vi "GetWindowInfo.vi"(8 "error in (no error)":errorcluster, 11 "Window Title (\"\")":string) -> (0 "error out":errorcluster, 1 "WINDOWINFO":T3 {"dwExStyle" format="%.0x"; "dwStyle" format="%.0x"}, 2 "Active?":bool, 3 "hWnd":T2, 4 "Window data":T1)   [LabVIEW 2011]
uses:
  hWnd.ctl
  window state.ctl
  user32.dll
panel:
  out "floating":bool
  out "maximized":bool
  out "minimized":bool
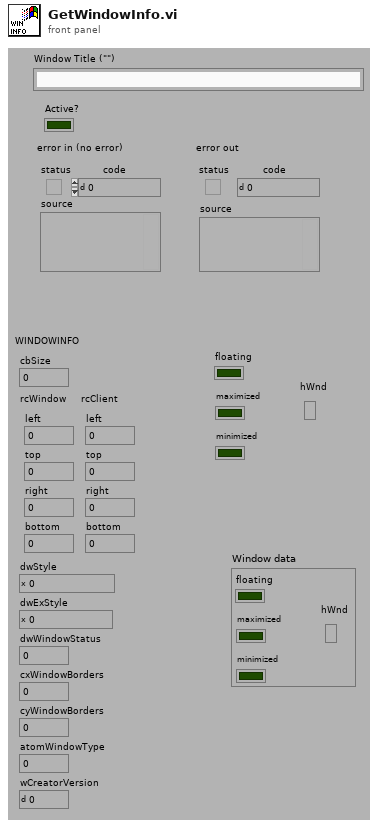
[diagram p1: front panel]
types:
  T1 = typedef "window state.ctl" = cluster{"minimized":bool, "maximized":bool, "floating":bool, "hWnd":T2}
  T2 = typedef "hWnd.ctl" = refnum<k1>
  T3 = cluster{"cbSize":i32, "rcWindow":cluster{"left":i32, "top":i32, "right":i32, "bottom":i32}, "rcClient":cluster{"left":i32, "top":i32, "right":i32, "bottom":i32}, "dwStyle":i32, "dwExStyle":i32, "dwWindowStatus":i32, "cxWindowBorders":u32, "cyWindowBorders":u32, "atomWindowType":u16, "wCreatorVersion":u16}
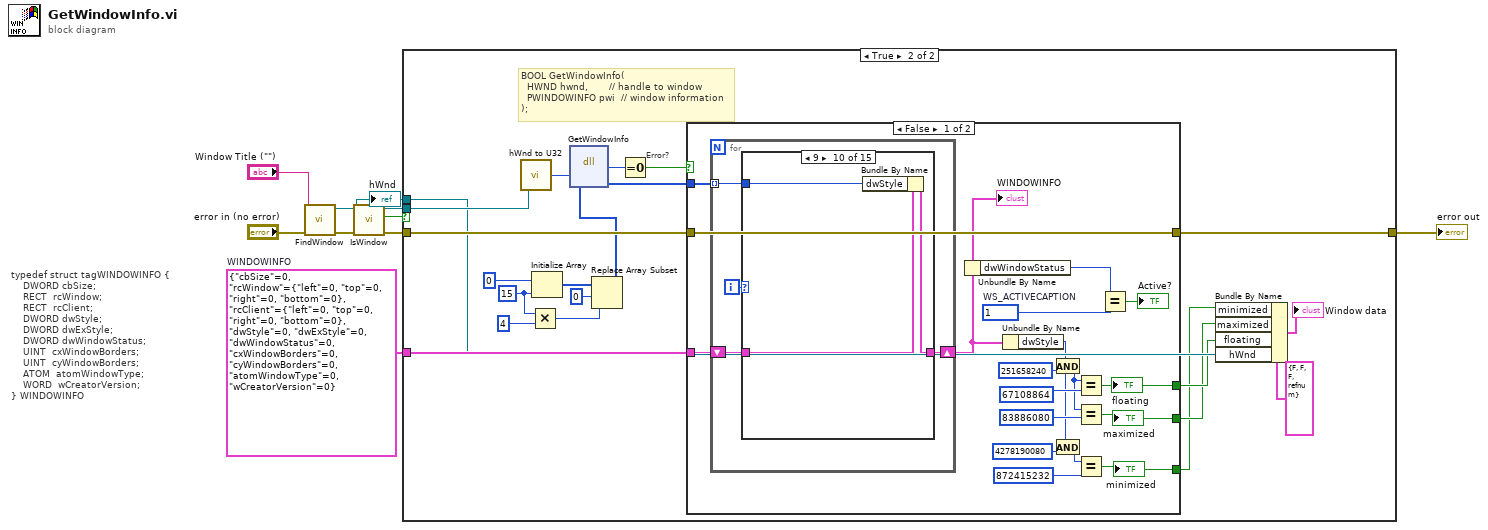
[diagram p0: block diagram]
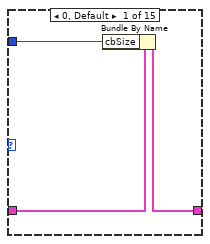
[diagram p3: hidden frame]
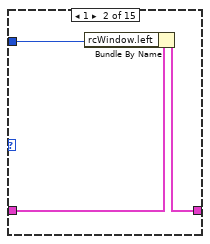
[diagram p4: hidden frame]
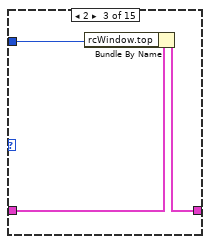
[diagram p5: hidden frame]
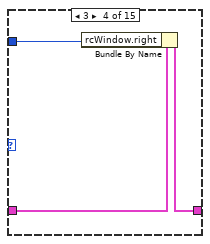
[diagram p6: hidden frame]
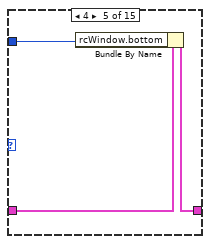
[diagram p7: hidden frame]
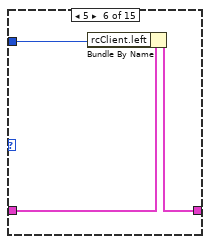
[diagram p8: hidden frame]
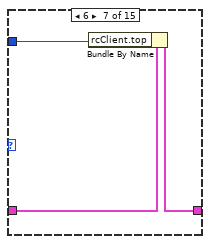
[diagram p9: hidden frame]
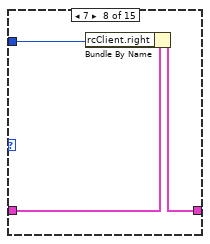
[diagram p10: hidden frame]
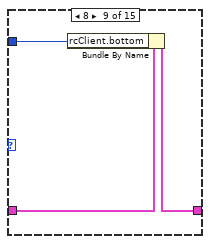
[diagram p11: hidden frame]
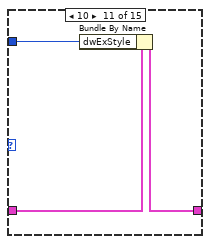
[diagram p12: hidden frame]
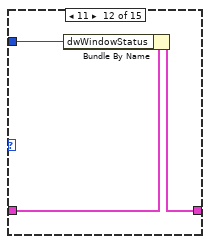
[diagram p13: hidden frame]
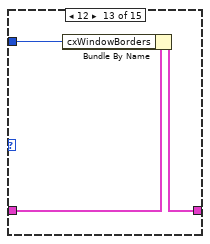
[diagram p14: hidden frame]
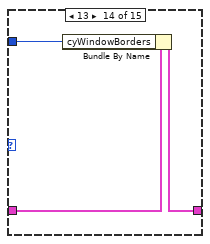
[diagram p15: hidden frame]
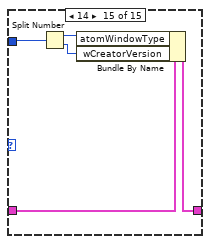
[diagram p16: hidden frame]
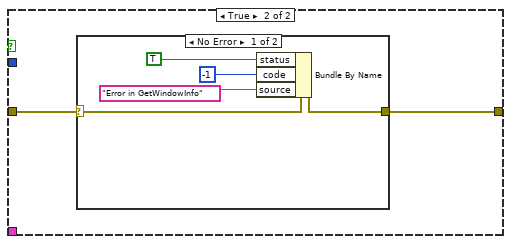
[diagram p17: hidden frame]
diagram:
  w3 = T3 {"cbSize"=0, "rcWindow"={"left"=0, "top"=0, "right"=0, "bottom"=0}, "rcClient"={"left"=0, "top"=0, "right"=0, "bottom"=0}, "dwStyle"=0, "dwExStyle"=0, "dwWindowStatus"=0, "cxWindowBorders"=0, "cyWindowBorders"=0, "atomWindowType"=0, "wCreatorVersion"=0}  # WINDOWINFO
  # "typedef struct tagWINDOWINFO {\n    DWORD cbSize;\n    RECT  rcWindow;\n    RECT  rcClient;\n    DWORD dwStyle;\n    DWORD dwExStyle;\n    DWORD dwWindowStatus;\n    UINT  cxWindowBorders;\n    UINT  cyWindowBorders;\n    ATOM  atomWindowType;\n    WORD  wCreatorVersion;\n} WINDOWINFO"
  n1 = call "FindWindow.vi"("error in (no error)"="error in (no error)", "window name (\"\")"="Window Title (\"\")") -> ("error out"=w7:errorcluster, "hWnd"=w1:T2)  [unwired: 6 out]
  "hWnd" <- w1
  n2 = call "IsWindow.vi"("error in (no error)"=w7, "hWnd (NULL)"=w1) -> ("error out"=w5:errorcluster, "Is Window?"=w6:bool, "dup hWnd"=w4:T2)  [unwired: 7 out]
  n3 = case shown="True" w6 {
    tunnel: w5 -> [w10 w26]
    tunnel: w4 -> [_ w31]
    tunnel: w3 -> [_ w23]
    tunnel: [w10 w25] -> w2
    tunnel: w1 -> [_ w14]
    frame False {
    }
    frame True {
      w22 = u32 15 ("dimension size")
      # "Error?"
      # "BOOL GetWindowInfo(\n  HWND hwnd,       // handle to window\n  PWINDOWINFO pwi  // window information\n);"
      n4 = call "hWnd to U32.vi"("hWnd"=w31) -> ("hWnd"=w30:u32)  [unwired: 4 out]
      n5 = Multiply(x=w22, y=u32 4) -> (x*y=w20:u32)
      n6 = Initialize Array(u32 0 ("dimension size"), w22) -> (w18:u32[])
      n7 = Replace Array Subset(array=w18, new element=w20, index=0) -> (w17:u32[])
      n8 = dll-call lib="User32.dll" fn="GetWindowInfo"("hwnd"=w30, "pwi"=w17) -> ("BOOL"=w28:i32, "pwi"=w29:u32[])  [unwired: 4 in, 2 out]
      n9 = Equal To 0?(x=w28) -> (x = 0?=w27:bool)
      n10 = case shown="False" w27 {
        tunnel: w29 -> [w44 _]
        tunnel: w26 -> [w46 w102]
        tunnel: [w46 w101] -> w25
        tunnel: w23 -> [w45 _]
        tunnel: [w34 _] -> w13
        tunnel: [w33 _] -> w12
        tunnel: [w32 _] -> w11
        frame False {
          w49 = 1  # WS_ACTIVECAPTION
          n11 = for {
            shift-right: [w50] -> w43
            shift-left: w45 -> [w51]
            tunnel: w44 -> [w53] mode=indexing
            i -> [w52]
            n12 = case shown="9" w52 {
              tunnel: w53 -> [w54 w57 w60 w63 w66 w69 w72 w75 w78 w81 w84 w87 w90 w93 w98]
              tunnel: w51 -> [w56 w59 w62 w65 w68 w71 w74 w77 w80 w83 w86 w89 w92 w95 w97]
              tunnel: [w55 w58 w61 w64 w67 w70 w73 w76 w79 w82 w85 w88 w91 w94 w96] -> w50
              frame 0, Default {
                n13 = Bundle By Name(cluster=w56, "cbSize"=w54) -> (w55:T3)
              }
              frame 1 {
                n14 = Bundle By Name(cluster=w59, "rcWindow.left"=w57) -> (w58:T3)
              }
              frame 2 {
                n15 = Bundle By Name(cluster=w62, "rcWindow.top"=w60) -> (w61:T3)
              }
              frame 3 {
                n16 = Bundle By Name(cluster=w65, "rcWindow.right"=w63) -> (w64:T3)
              }
              frame 4 {
                n17 = Bundle By Name(cluster=w68, "rcWindow.bottom"=w66) -> (w67:T3)
              }
              frame 5 {
                n18 = Bundle By Name(cluster=w71, "rcClient.left"=w69) -> (w70:T3)
              }
              frame 6 {
                n19 = Bundle By Name(cluster=w74, "rcClient.top"=w72) -> (w73:T3)
              }
              frame 7 {
                n20 = Bundle By Name(cluster=w77, "rcClient.right"=w75) -> (w76:T3)
              }
              frame 8 {
                n21 = Bundle By Name(cluster=w80, "rcClient.bottom"=w78) -> (w79:T3)
              }
              frame 9 {
                n22 = Bundle By Name(cluster=w83, "dwStyle"=w81) -> (w82:T3)
              }
              frame 10 {
                n23 = Bundle By Name(cluster=w86, "dwExStyle"=w84) -> (w85:T3)
              }
              frame 11 {
                n24 = Bundle By Name(cluster=w89, "dwWindowStatus"=w87) -> (w88:T3)
              }
              frame 12 {
                n25 = Bundle By Name(cluster=w92, "cxWindowBorders"=w90) -> (w91:T3)
              }
              frame 13 {
                n26 = Bundle By Name(cluster=w95, "cyWindowBorders"=w93) -> (w94:T3)
              }
              frame 14 {
                n27 = Split Number(x=w98) -> (hi(x)=w100:u16, lo(x)=w99:u16)
                n28 = Bundle By Name(cluster=w97, "atomWindowType"=w100, "wCreatorVersion"=w99) -> (w96:T3)
              }
            }
          }
          "WINDOWINFO" <- w43
          n29 = Unbundle By Name(w43) -> ("dwWindowStatus"=w48:i32)
          n30 = Unbundle By Name(w43) -> ("dwStyle"=w35:i32)
          n31 = And(x=w35, y=u32 251658240) -> (x .and. y?=w38:u32)
          n32 = And(x=w35, y=u32 4278190080) -> (x .and. y?=w40:u32)
          n33 = Equal?(x=w38, y=u32 67108864) -> (x = y?=w34:bool)
          "floating" <- w34
          n34 = Equal?(x=w38, y=u32 83886080) -> (x = y?=w33:bool)
          "maximized" <- w33
          n35 = Equal?(x=w40, y=u32 872415232) -> (x = y?=w32:bool)
          "minimized" <- w32
          n36 = Equal?(x=w48, y=w49) -> (x = y?=→"Active?":bool)
        }
        frame True {
          n37 = case shown="No Error" w102 {
            selector: w102 -> [w107 w108]
            tunnel: [w106 w108] -> w101
            frame No Error {
              n38 = Bundle By Name(cluster=w107, "status"=TRUE, "code"=-1, "source"="Error in GetWindowInfo") -> (w106:errorcluster)
            }
            frame Error {
            }
          }
        }
      }
      n39 = Bundle By Name(cluster=T1 {"minimized"=FALSE, "maximized"=FALSE, "floating"=FALSE, "hWnd"=refnum} ("Window data"), "minimized"=w11, "maximized"=w12, "floating"=w13, "hWnd"=w14) -> (→"Window data":T1)
    }
  }
  "error out" <- w2
